vi "LSX Set EEP Rom Value.vi"(8 "error in (no error)":errorcluster, 9 "Value":u8, 10 "Offset":u8, 11 "lLSID":i32) -> (0 "error out":errorcluster, 3 "function return":i32)   [LabVIEW 2016, in "Tango_DLL.lvlib"]
doc: "TANGOAPI int TANGOCALL LSX_SetEEPRomValue (int lLSID, byte Offset, byte Value);"
uses:
  Tango_DLL.lvlib
  2017/Microscope Control/Device Library/Stages/Marzhauser/SCAN IM 120 x 80/Tango DLL VIs/Tango_DLL.dll
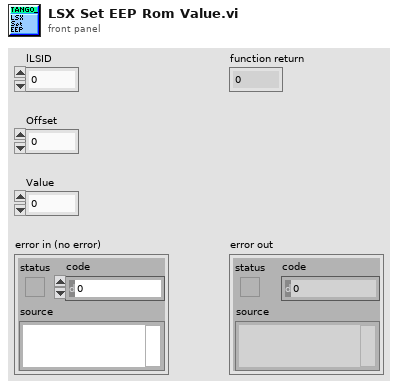
[diagram p1: front panel]
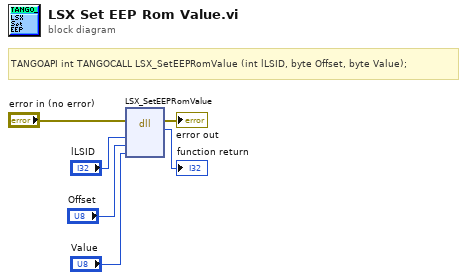
[diagram p0: block diagram]
diagram:
  # "TANGOAPI int TANGOCALL LSX_SetEEPRomValue (int lLSID, byte Offset, byte Value);"
  n1 = dll-call lib="C:/Users/4PiSMS/Documents/Microscope Control/2017/Microscope Control/Device Library/Stages/Marzhauser/SCAN IM 120 x 80/Tango DLL VIs/Tango_DLL.*" fn="LSX_SetEEPRomValue"(error in="error in (no error)", "lLSID"="lLSID", "Offset"="Offset", "Value"="Value") -> (error out=→"error out":errorcluster, →"function return":i32)  [unwired: 5 in, 1 out]
